vi "Read Offset Values.vi"(6 "error in":errorcluster, 8 "MaxRead":i32, 9 "Channel in":u16) -> (0 "error out":errorcluster, 1 "Messages":T2(array[cluster]) {"ID" format="%.0x"; "DATA[0]" format="%.0x"; "DATA[1]" format="%.0x"; "DATA[2]" format="%.0x"; "DATA[3]" format="%.0x"; "DATA[4]" format="%.0x"; "DATA[5]" format="%.0x"; "DATA[6]" format="%.0x"; "DATA[7]" format="%.0x"}, 2 "Pass":bool, 3 "Channel out":u16)   [LabVIEW 2023]
uses:
  4f930f32-d09a-43ef-bca1-8b214b378bd5.vi
  e8470de1-fa2d-4ee3-b50e-96bd89dc731f.vi
  Communication/PCAN2023/PCAN API.lvlib
panel:
  out "MessageBuffer out 4":T1 {"ID" format="%.0x"; "DATA[0]" format="%.0x"; "DATA[1]" format="%.0x"; "DATA[2]" format="%.0x"; "DATA[3]" format="%.0x"; "DATA[4]" format="%.0x"; "DATA[5]" format="%.0x"; "DATA[6]" format="%.0x"; "DATA[7]" format="%.0x"}
  in  "stop 4":bool
  out "Numeric 4":i32
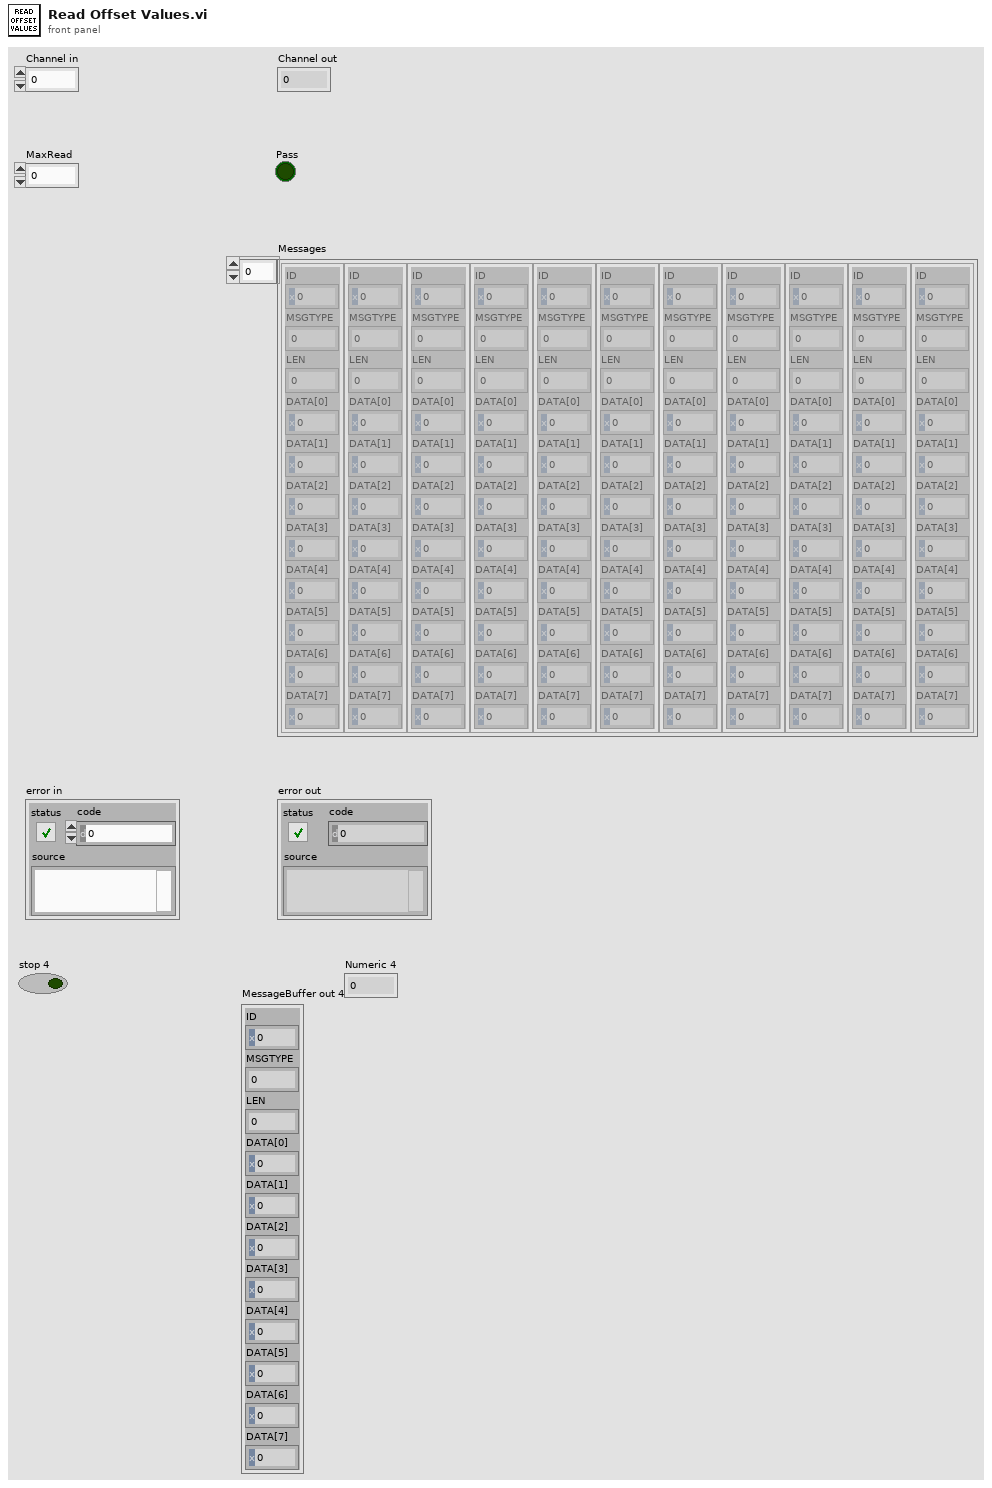
[diagram p1: front panel]
types:
  T1 = cluster{"ID":u32, "MSGTYPE":u8, "LEN":u8, "DATA[0]":u8, "DATA[1]":u8, "DATA[2]":u8, "DATA[3]":u8, "DATA[4]":u8, "DATA[5]":u8, "DATA[6]":u8, "DATA[7]":u8}
  T2 = cluster{"ID":u32, "MSGTYPE":u8, "LEN":u8, "DATA[0]":u8, "DATA[1]":u8, "DATA[2]":u8, "DATA[3]":u8, "DATA[4]":u8, "DATA[5]":u8, "DATA[6]":u8, "DATA[7]":u8}[]
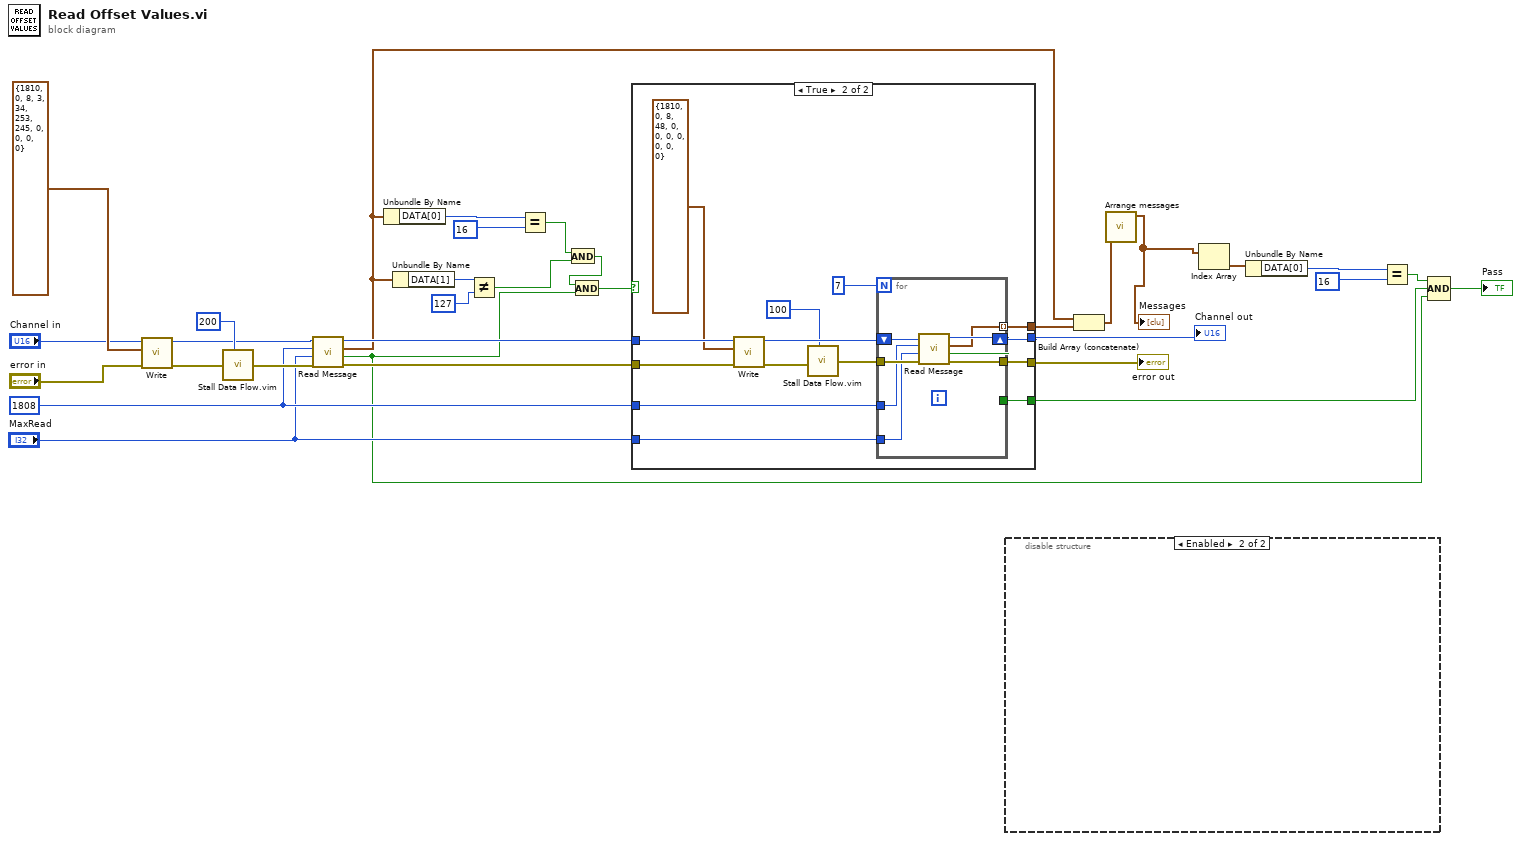
[diagram p0: block diagram]
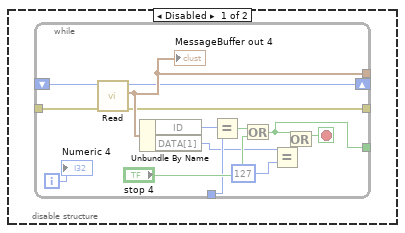
[diagram p2: hidden frame]
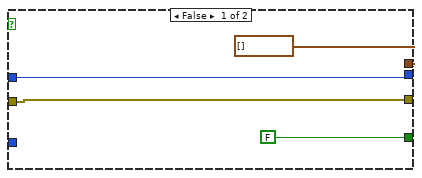
[diagram p3: hidden frame]
diagram:
  (unwired) u32 200 ("milliseconds to wait")
  w13 = u32 1808 ("ID")
  n1 = call "Write.vi"("error in"="error in", "MessageBuffer"=T1 {"ID"=1810, "MSGTYPE"=0, "LEN"=8, "DATA[0]"=3, "DATA[1]"=34, "DATA[2]"=253, "DATA[3]"=245, "DATA[4]"=0, "DATA[5]"=0, "DATA[6]"=0, "DATA[7]"=0}, "Channel"="Channel in") -> ("error out"=w27:errorcluster, "Channel out"=w17:u16)  [unwired: 5 in, 2 out]
  n2 = call "Stall Data Flow.vim"("value in"=w27, "milliseconds to wait"=u32 200) -> ("value out"=w16:errorcluster)  [unwired: 1 out]
  n3 = call "Read Message.vi"("error in"=w16, "MaxRead"="MaxRead", "ID"=w13, "Channel in"=w17) -> ("error out"=w14:errorcluster, "Passed"=w10:bool, "Last Message"=w7:T1, "Channel out"=w15:u16)  [unwired: 3 in, 1 out]
  n4 = Unbundle By Name(w7) -> ("DATA[0]"=w9:u8)
  n5 = Unbundle By Name(w7) -> ("DATA[1]"=w20:u8)
  n6 = Not Equal?(x=w20, y=u8 127) -> (x != y?=w5:bool)
  n7 = Equal?(x=w9, y=u8 16) -> (x = y?=w6:bool)
  n8 = And(x=w6, y=w5) -> (x .and. y?=w4:bool)
  n9 = And(x=w4, y=w10) -> (x .and. y?=w11:bool)
  n10 = case shown="True" w11 {
    tunnel: w15 -> [w35 w50]
    tunnel: w14 -> [w34 w49]
    tunnel: [w34 w48] -> w24
    tunnel: [FALSE w47] -> w23
    tunnel: [w35 w45] -> w22
    tunnel: [T2 [] w39] -> w21
    tunnel: w13 -> [_ w38]
    tunnel: "MaxRead" -> [_ w37]
    frame False {
    }
    frame True {
      n11 = call "Write.vi"("error in"=w49, "MessageBuffer"=T1 {"ID"=1810, "MSGTYPE"=0, "LEN"=8, "DATA[0]"=48, "DATA[1]"=0, "DATA[2]"=0, "DATA[3]"=0, "DATA[4]"=0, "DATA[5]"=0, "DATA[6]"=0, "DATA[7]"=0}, "Channel"=w50) -> ("error out"=w42:errorcluster, "Channel out"=w46:u16)  [unwired: 5 in, 2 out]
      n12 = call "Stall Data Flow.vim"("value in"=w42, "milliseconds to wait"=u32 100) -> ("value out"=w44:errorcluster)  [unwired: 1 out]
      n13 = for {
        N: 7 -> [_]
        tunnel: [w54] -> w47
        shift-right: [w56] -> w45
        shift-left: w46 -> [w58]
        tunnel: [w55] -> w39 mode=indexing
        tunnel: w44 -> [w57]
        tunnel: [w53] -> w48
        tunnel: w38 -> [w52]
        tunnel: w37 -> [w51]
        n14 = call "Read Message.vi"("error in"=w57, "MaxRead"=w51, "ID"=w52, "Channel in"=w58) -> ("error out"=w53:errorcluster, "Passed"=w54:bool, "Last Message"=w55:T1, "Channel out"=w56:u16)  [unwired: 3 in, 1 out]
      }
    }
  }
  "error out" <- w24
  "Channel out" <- w22
  n15 = disable-structure shown="Enabled" {
    frame Disabled {
      n16 = while {
        tunnel: _ -> [w73]
        tunnel: _ -> [w68]
        tunnel: [w67] -> _
        tunnel: [w66] -> _
        tunnel: [w59] -> _
        shift-right: [w64] -> _
        shift-left: _ -> [w65]
        i -> [w69]
        stop <- w61 stop-if-true
        n17 = call "Read.vi"("error in"=w73, "Channel"=w65) -> ("error out"=w66:errorcluster, "MessageBuffer out"=w67:T1, "Channel out"=w64:u16)  [unwired: 6 in, 1 out]
        "MessageBuffer out 4" <- w67
        n18 = Unbundle By Name(w67) -> ("ID"=w72:u32, "DATA[1]"=w62:u8)
        n19 = Equal?(x=w72, y=w68) -> (x = y?=w71:bool)
        n20 = Or(x=w71, y="stop 4") -> (x .or. y?=w59:bool)
        n21 = Equal?(x=w62, y=u8 127) -> (x = y?=w60:bool)
        n22 = Or(x=w59, y=w60) -> (x .or. y?=w61:bool)
        "Numeric 4" <- w69
      }
    }
    frame Enabled {
    }
  }
  n23 = Build Array (concatenate)(w7, w21) -> (w3:T2)
  n24 = call "Arrange messages.vi"("Array in"=w3) -> ("Array out"=w2:T2)  [unwired: 10 in]
  "Messages" <- w2
  n25 = Index Array(array=w2) -> (element=w1:T1)  [unwired: 1 in]
  n26 = Unbundle By Name(w1) -> ("DATA[0]"=w26:u8)
  n27 = Equal?(x=w26, y=u8 16) -> (x = y?=w18:bool)
  n28 = Compound Arithmetic op=AND(w18, w23, w10) -> (→"Pass":bool)
